vi "myRIO-1900 Quadrotor FPGA.vi"() -> ()   [LabVIEW 2013]
uses:
  <vilib>/Platform/TimedLoop/XDataNode/timing_clust.ctl
  <vilib>/Platform/TimedLoop/XDataNode/nitl_modes.ctl
  <vilib>/Platform/TimedLoop/XDataNode/wakeup.ctl
  <vilib>/rvi/Emulation/niFpgaSctlEmulationGetInTimedLoop.vi
  <vilib>/rvi/Emulation/niFpgaEmulationReportErrorSimple.vi
  <vilib>/rvi/Emulation/niFpgaGetClockAttributes.vi
  <vilib>/rvi/Emulation/niFpgaCriticalErrorInLSC.vi
  <vilib>/rvi/eio/common/nirviEmuTemplateMethod_errors.vi
  <vilib>/rvi/Emulation/niFpgaProcessEmulError.vi
  <vilib>/Platform/TimedLoop/XDataNode/XDataNode.xnode
  <vilib>/eio/EIOMethodNode/EIOMethodNode.xnode
  <vilib>/Platform/TimedLoop/XDataNode/XDNodeRunTimeDep.lvlib
panel:
  in  "FeedDog":bool
  in  "CounterMAX":u32
  in  "PWM1":u16
  in  "PWM2":u16
  in  "PWM0":u16
  in  "PWM3":u16
  in  "MotorEn":bool
  in  "PWMOutputEN":bool
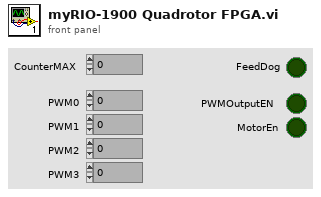
[diagram p1: front panel]
types:
  T1 = cluster{"PWM0":refnum<k21>, "PWM1":refnum<k21>, "PWM2":refnum<k21>, "PWM3":refnum<k21>}
  T2 = typedef "XDNodeRunTimeDep.lvlib/timing_clust.ctl" = cluster{"Expected End [f-1]":u64, "Actual End [f-1]":u64, "Finished Late? [f-1]":bool, "Expected End [i-1]":u64, "Actual End [i-1]":u64, "Finished Late? [i-1]":bool, "Expected Start [i]":u64, "Actual Start [i]":u64, "Expected Start [f]":u64, "Actual Start [f]":u64, "Source Name":string, "Structure Name":string, "Period":i64, "Deadline":i64, "Offset":i64, "Start":i64, "Priority":i32, "Timeout":i32, "Mode":T3, "Wakeup Reason":T4, "Error":errorcluster, "Source Type":string, "Secondary Source Type":string, "Global End Time":u64, "Global Start Time":u64, "Frame Duration":u64, "Iteration Duration":u64, "Assigned CPU":i32, "I/O Scan Engine Mode":u32}
  T3 = typedef "XDNodeRunTimeDep.lvlib/nitl_modes.ctl" = enum32{"No Change", "Process missed periods, maintain original phase", "Discard missed periods, maintain original phase", "Process missed periods, ignore original phase", "Discard missed periods, ignore original phase"}
  T4 = typedef "XDNodeRunTimeDep.lvlib/wakeup.ctl" = enum32{"Normal", "Aborted", "Asynchronous wakeup", "Timing source error", "Timed loop error", "Timeout"}
  T5 = cluster{"NextState":enum8{"OutputEN", "GetInput", "Update", "CycleOver"}, "PWMCnt0":u16, "PWMCnt1":u16, "PWMCnt2":u16, "PWMCnt3":u16, "Counter":u32, "WatchDog":u32, "TimeOut?":bool, "CounterMAX":u32}
  T6 = enum8{"OutputEN", "GetInput", "Update", "CycleOver"}
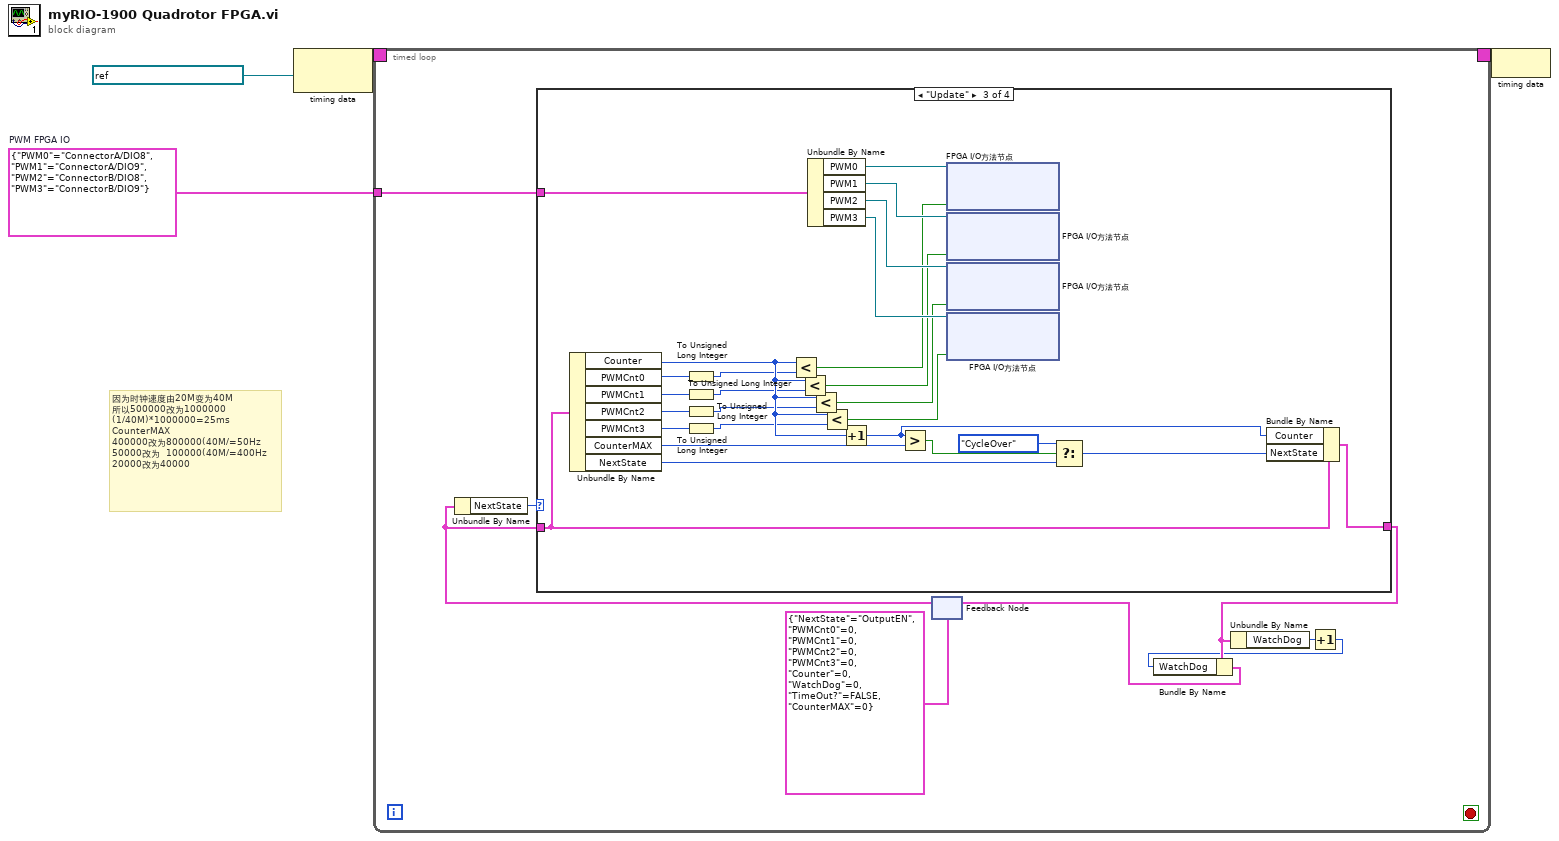
[diagram p0: block diagram]
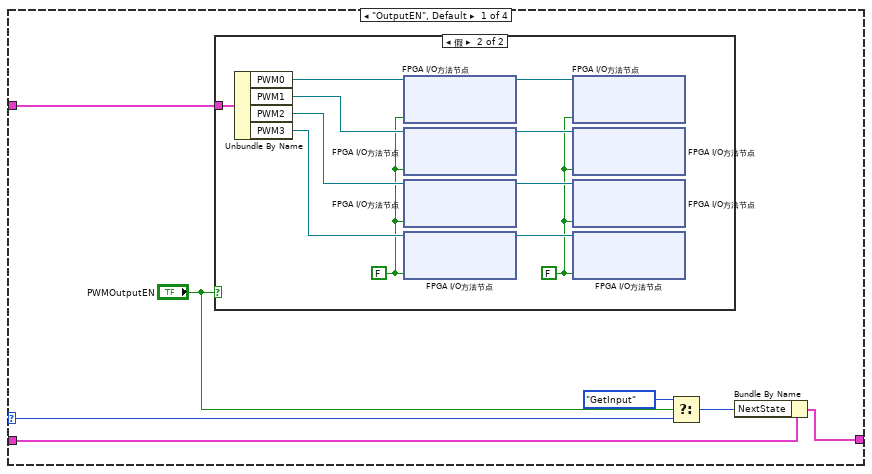
[diagram p2: hidden frame]
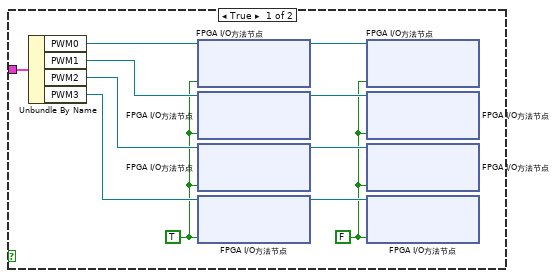
[diagram p3: hidden frame]
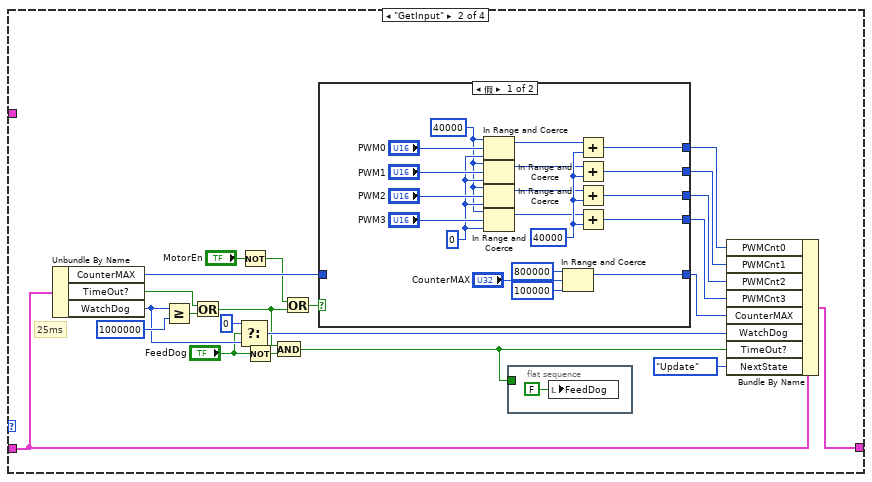
[diagram p4: hidden frame]
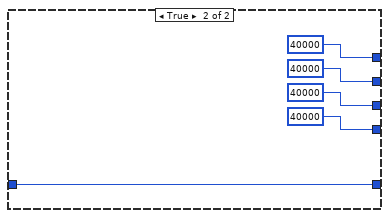
[diagram p5: hidden frame]
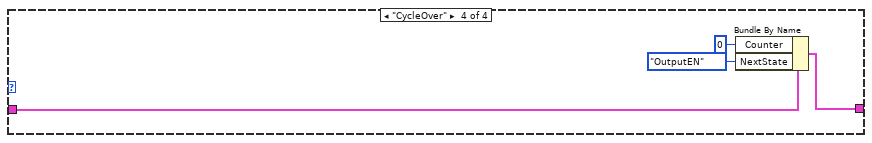
[diagram p6: hidden frame]
diagram:
  w2 = T1 {"PWM0"="ConnectorA/DIO8", "PWM1"="ConnectorA/DIO9", "PWM2"="ConnectorB/DIO8", "PWM3"="ConnectorB/DIO9"}  # PWM FPGA IO
  # "因为时钟速度由20M变为40M\n所以500000改为1000000\n(1/40M)*1000000=25ms\nCounterMAX\n400000改为800000(40M/=50Hz\n50000改为  100000(40M/=400Hz\n20000改为40000"
  n1 = node-c288(refnum<k21> "40 MHz Onboard Clock" ("源名称")) -> (w4:T2)
  n2 = timed-loop {
    timing: w4 -> [_]
    timing-out: [_] -> w3
    tunnel: w2 -> [w9]
    stop <- _ stop-if-true
    n3 = feedback #1(T5 {"NextState"=enum."OutputEN", "PWMCnt0"=0, "PWMCnt1"=0, "PWMCnt2"=0, "PWMCnt3"=0, "Counter"=0, "WatchDog"=0, "TimeOut?"=FALSE, "CounterMAX"=0}) -> (w11:T5)
    n4 = Unbundle By Name(w11) -> ("NextState"=w10:T6)
    n5 = case shown="\"Update\"" w10 {
      selector: w10 -> [w15 _ _ _]
      tunnel: w11 -> [w18 w62 w97 w118]
      tunnel: [w17 w63 w96 w117] -> w8
      tunnel: w9 -> [w19 _ w110 _]
      frame "OutputEN", Default {
        n6 = case shown="假" "PWMOutputEN" {
          tunnel: w19 -> [w30 w41]
          frame True {
            w20 = FALSE ("启用")
            w25 = TRUE ("启用")
            n7 = Unbundle By Name(w30) -> ("PWM0"=w29:refnum<k21>, "PWM1"=w26:refnum<k21>, "PWM2"=w28:refnum<k21>, "PWM3"=w27:refnum<k21>)
            n8 = xnode "FPGA I/O方法节点"("FPGA I/O In"=w29, "启用"=w25) -> ("FPGA I/O Out"=w24:refnum<k21>)
            n9 = xnode "FPGA I/O方法节点"("FPGA I/O In"=w26, "启用"=w25) -> ("FPGA I/O Out"=w23:refnum<k21>)
            n10 = xnode "FPGA I/O方法节点"("FPGA I/O In"=w28, "启用"=w25) -> ("FPGA I/O Out"=w22:refnum<k21>)
            n11 = xnode "FPGA I/O方法节点"("FPGA I/O In"=w27, "启用"=w25) -> ("FPGA I/O Out"=w21:refnum<k21>)
            n12 = xnode "FPGA I/O方法节点"("FPGA I/O In"=w24, "数据"=w20) -> ()  [unwired: 1 out]
            n13 = xnode "FPGA I/O方法节点"("FPGA I/O In"=w23, "数据"=w20) -> ()  [unwired: 1 out]
            n14 = xnode "FPGA I/O方法节点"("FPGA I/O In"=w22, "数据"=w20) -> ()  [unwired: 1 out]
            n15 = xnode "FPGA I/O方法节点"("FPGA I/O In"=w21, "数据"=w20) -> ()  [unwired: 1 out]
          }
          frame False {
            w31 = FALSE ("启用")
            w36 = FALSE ("启用")
            n16 = Unbundle By Name(w41) -> ("PWM0"=w40:refnum<k21>, "PWM1"=w37:refnum<k21>, "PWM2"=w39:refnum<k21>, "PWM3"=w38:refnum<k21>)
            n17 = xnode "FPGA I/O方法节点"("FPGA I/O In"=w40, "启用"=w36) -> ("FPGA I/O Out"=w35:refnum<k21>)
            n18 = xnode "FPGA I/O方法节点"("FPGA I/O In"=w37, "启用"=w36) -> ("FPGA I/O Out"=w34:refnum<k21>)
            n19 = xnode "FPGA I/O方法节点"("FPGA I/O In"=w39, "启用"=w36) -> ("FPGA I/O Out"=w33:refnum<k21>)
            n20 = xnode "FPGA I/O方法节点"("FPGA I/O In"=w38, "启用"=w36) -> ("FPGA I/O Out"=w32:refnum<k21>)
            n21 = xnode "FPGA I/O方法节点"("FPGA I/O In"=w35, "数据"=w31) -> ()  [unwired: 1 out]
            n22 = xnode "FPGA I/O方法节点"("FPGA I/O In"=w34, "数据"=w31) -> ()  [unwired: 1 out]
            n23 = xnode "FPGA I/O方法节点"("FPGA I/O In"=w33, "数据"=w31) -> ()  [unwired: 1 out]
            n24 = xnode "FPGA I/O方法节点"("FPGA I/O In"=w32, "数据"=w31) -> ()  [unwired: 1 out]
          }
        }
        n25 = Select(t=T6."GetInput", s="PWMOutputEN", f=w15) -> (s? t:f=w14:T6)
        n26 = Bundle By Name(cluster=w18, "NextState"=w14) -> (w17:T5)
      }
      frame "GetInput" {
        # "25ms"
        n27 = Unbundle By Name(w62) -> ("CounterMAX"=w46:u32, "TimeOut?"=w59:bool, "WatchDog"=w57:u32)
        n28 = Greater Or Equal?(x=w57, y=u32 1000000) -> (x >= y?=w60:bool)
        n29 = Or(x=w59, y=w60) -> (x .or. y?=w43:bool)
        n30 = Select(t=u32 0, s="FeedDog", f=w57) -> (s? t:f=w58:u32)
        n31 = Not(x="MotorEn") -> (.not. x?=w42:bool)
        n32 = Not(x="FeedDog") -> (.not. x?=w54:bool)
        n33 = And(x=w43, y=w54) -> (x .and. y?=w47:bool)
        n34 = Or(x=w42, y=w43) -> (x .or. y?=w44:bool)
        n35 = case shown="假" w44 {
          tunnel: [w78 u16 40000 ("PWM0")] -> w53
          tunnel: [w77 u16 40000 ("PWM1")] -> w52
          tunnel: [w76 u16 40000 ("PWM2")] -> w51
          tunnel: [w75 u16 40000 ("PWM3")] -> w50
          tunnel: [w80 w85] -> w49
          tunnel: w46 -> [_ w85]
          frame False {
            w70 = u16 0 ("PWM1")
            w69 = u16 40000 ("PWM1")
            w79 = u16 40000
            n36 = In Range and Coerce(upper limit=w69, x="PWM0", lower limit=w70) -> (coerced(x)=w68:u16)  [unwired: 1 out]
            n37 = In Range and Coerce(upper limit=w69, x="PWM1", lower limit=w70) -> (coerced(x)=w67:u16)  [unwired: 1 out]
            n38 = In Range and Coerce(upper limit=w69, x="PWM2", lower limit=w70) -> (coerced(x)=w66:u16)  [unwired: 1 out]
            n39 = In Range and Coerce(upper limit=w69, x="PWM3", lower limit=w70) -> (coerced(x)=w65:u16)  [unwired: 1 out]
            n40 = In Range and Coerce(upper limit=u32 800000 ("上限"), x="CounterMAX", lower limit=u32 100000 ("下限")) -> (coerced(x)=w80:u32)  [unwired: 1 out]
            n41 = Add(x=w68, y=w79) -> (x+y=w78:u16)
            n42 = Add(x=w67, y=w79) -> (x+y=w77:u16)
            n43 = Add(x=w66, y=w79) -> (x+y=w76:u16)
            n44 = Add(x=w65, y=w79) -> (x+y=w75:u16)
          }
          frame True {
          }
        }
        n45 = flat-sequence {
          tunnel: w47 -> [_]
          frame #0 {
            n46 = local write "FeedDog"(FALSE ("FeedDog")) -> ()
          }
        }
        n47 = Bundle By Name(cluster=w62, "PWMCnt0"=w53, "PWMCnt1"=w52, "PWMCnt2"=w51, "PWMCnt3"=w50, "CounterMAX"=w49, "WatchDog"=w58, "TimeOut?"=w47, "NextState"=T6."Update") -> (w63:T5)
      }
      frame "Update" {
        n48 = Unbundle By Name(w97) -> ("Counter"=w101:u32, "PWMCnt0"=w114:u16, "PWMCnt1"=w113:u16, "PWMCnt2"=w112:u16, "PWMCnt3"=w111:u16, "CounterMAX"=w100:u32, "NextState"=w98:T6)
        n49 = To Unsigned Long Integer(number=w114) -> (unsigned 32bit integer=w92:u32)
        n50 = To Unsigned Long Integer(number=w113) -> (unsigned 32bit integer=w91:u32)
        n51 = To Unsigned Long Integer(number=w112) -> (unsigned 32bit integer=w90:u32)
        n52 = To Unsigned Long Integer(number=w111) -> (unsigned 32bit integer=w89:u32)
        n53 = Less?(x=w101, y=w92) -> (x < y?=w105:bool)
        n54 = Less?(x=w101, y=w91) -> (x < y?=w104:bool)
        n55 = Unbundle By Name(w110) -> ("PWM0"=w109:refnum<k21>, "PWM1"=w108:refnum<k21>, "PWM2"=w107:refnum<k21>, "PWM3"=w106:refnum<k21>)
        n56 = Less?(x=w101, y=w90) -> (x < y?=w103:bool)
        n57 = Less?(x=w101, y=w89) -> (x < y?=w102:bool)
        n58 = Increment(x=w101) -> (x+1=w93:u32)
        n59 = Greater?(x=w93, y=w100) -> (0:w99:bool)
        n60 = xnode "FPGA I/O方法节点"("FPGA I/O In"=w109, "数据"=w105) -> ()  [unwired: 1 out]
        n61 = xnode "FPGA I/O方法节点"("FPGA I/O In"=w108, "数据"=w104) -> ()  [unwired: 1 out]
        n62 = xnode "FPGA I/O方法节点"("FPGA I/O In"=w107, "数据"=w103) -> ()  [unwired: 1 out]
        n63 = xnode "FPGA I/O方法节点"("FPGA I/O In"=w106, "数据"=w102) -> ()  [unwired: 1 out]
        n64 = Select(t=T6."CycleOver", s=w99, f=w98) -> (s? t:f=w95:T6)
        n65 = Bundle By Name(cluster=w97, "Counter"=w93, "NextState"=w95) -> (w96:T5)
      }
      frame "CycleOver" {
        n66 = Bundle By Name(cluster=w118, "Counter"=u32 0, "NextState"=T6."OutputEN") -> (w117:T5)
      }
    }
    n67 = Unbundle By Name(w8) -> ("WatchDog"=w7:u32)
    n68 = Increment(x=w7) -> (x+1=w6:u32)
    n69 = Bundle By Name(cluster=w8, "WatchDog"=w6) -> (w5:T5)
    n70 = feedback-in #1(w5) -> ()
  }
  n71 = node-c288(w3) -> ()
